vi "intelligencia.vi"   [LabVIEW 2015]
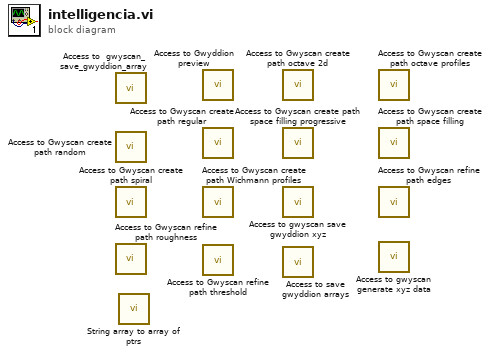
[diagram p0: block diagram]
diagram:
  n1 = call <userlib>:"Access to  gwyscan_save_gwyddion_array.vi"() -> ()  [unwired: 11 in, 1 out]
  n2 = call <userlib>:"Access to Gwyscan create path random.vi"() -> ()  [unwired: 8 in, 4 out]
  n3 = call <userlib>:"Access to Gwyscan create path spiral.vi"() -> ()  [unwired: 7 in, 5 out]
  n4 = call <userlib>:"Access to Gwyscan refine path roughness.vi"() -> ()  [unwired: 4 in, 5 out]
  n5 = call <userlib>:"String array to array of ptrs.vi"() -> ()  [unwired: 3 in, 3 out]
  n6 = call <userlib>:"Access to Gwyddion preview.vi"() -> ()  [unwired: 10 in, 2 out]
  n7 = call <userlib>:"Access to Gwyscan create path regular.vi"() -> ()  [unwired: 8 in, 4 out]
  n8 = call <userlib>:"Access to Gwyscan create path Wichmann profiles.vi"() -> ()  [unwired: 7 in, 5 out]
  n9 = call <userlib>:"Access to Gwyscan refine path threshold.vi"() -> ()  [unwired: 5 in, 7 out]
  n10 = call <userlib>:"Access to Gwyscan create path octave 2d.vi"() -> ()  [unwired: 8 in, 4 out]
  n11 = call <userlib>:"Access to Gwyscan create path space filling progressive.vi"() -> ()  [unwired: 8 in, 4 out]
  n12 = call <userlib>:"Access to gwyscan save gwyddion xyz.vi"() -> ()  [unwired: 11 in, 1 out]
  n13 = call <userlib>:"Access to save gwyddion arrays.vi"() -> ()  [unwired: 5 in, 1 out]
  n14 = call <userlib>:"Access to Gwyscan create path octave profiles.vi"() -> ()  [unwired: 8 in, 4 out]
  n15 = call <userlib>:"Access to Gwyscan create path space filling.vi"() -> ()  [unwired: 8 in, 4 out]
  n16 = call <userlib>:"Access to Gwyscan refine path edges.vi"() -> ()  [unwired: 7 in, 5 out]
  n17 = call <userlib>:"Access to gwyscan generate xyz data.vi"() -> ()  [unwired: 4 in, 3 out]
